vi "tm3samp_09_masterpulse_sequence.vi"() -> ()   [LabVIEW 2011]
panel:
  in  "Interval":dbl=0.5
  out "DCAM Version":string
  out "Library Version":string
  out "Image":u16[][](graph)
  out "Frames Per Second":dbl
  in  "Quit":bool
  out "Error Out":errorcluster {"code" format="%.0x"}
  # "This example will demonstrate how to configure the master pulse and use it for internal trigger capture.  The master pulse signal is also sent to the output trigger in this example."
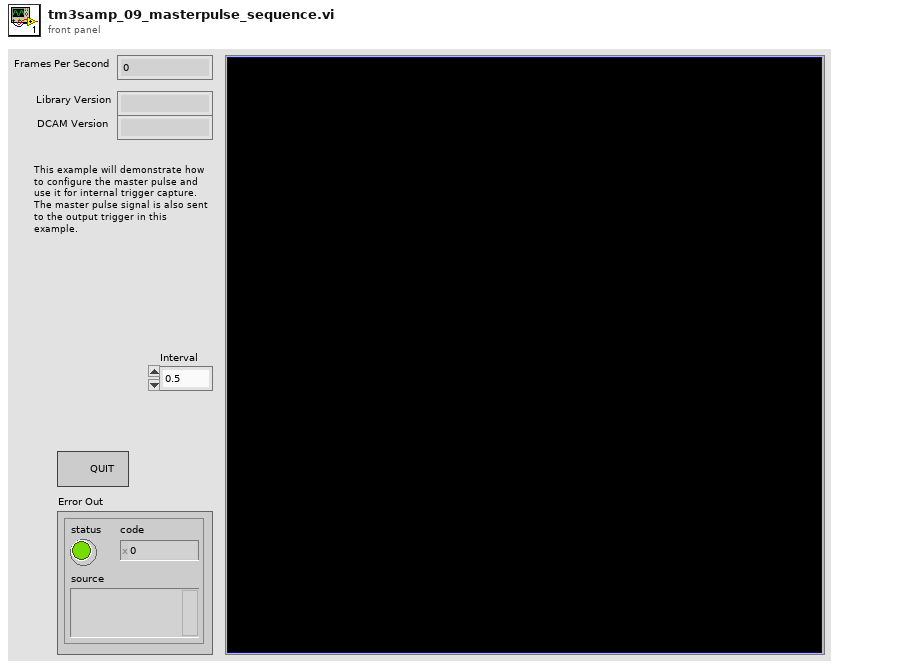
[diagram p1: front panel]
types:
  T1 = cluster{"Capture Library":string, "DCAM-API":string}
  T2 = cluster{"Mode":u32, "Polarity":u32, "Period":dbl, "Delay":dbl}
  T3 = cluster{"Mode":u32, "Source":u32, "Interval":dbl, "Burst":u32}
  T4 = cluster{"height":u32, "width":u32, "datatype":u32}
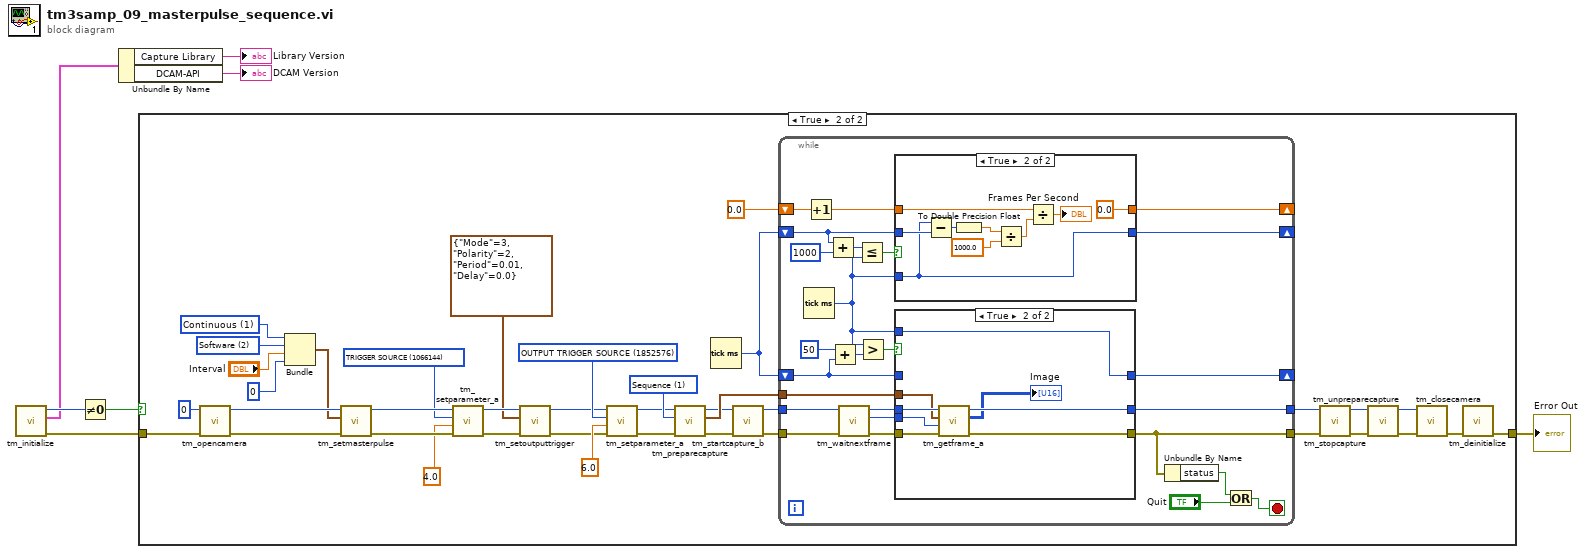
[diagram p0: block diagram]
diagram:
  n1 = call <userlib>:"tm_initialize.vi"() -> ("error out"=w4:errorcluster, "Version Info"=w3:T1, "Number Of Cameras"=w5:u32)  [unwired: 8 in, 1 out]
  n2 = Not Equal To 0?(x=w5) -> (x != 0?=w7:bool)
  n3 = Unbundle By Name(w3) -> ("Capture Library"=→"Library Version":string, "DCAM-API"=→"DCAM Version":string)
  n4 = case shown="True" w7 {
    tunnel: w4 -> [w8 w46]
    tunnel: [w8 w43] -> w6
    frame False {
    }
    frame True {
      w17 = u32 1852576 items=["SENSOR MODE"=4212128, "CCD MODE"=4212384, "READOUT MODE"=4211872, "ACTIVE VIEW INDEX"=4343136, "BITS PER CHANNEL"=4342976, "IMAGE PIXEL TYPE"=4343296, "BINNING"=4215968, "EXPOSURE TIME"=2049184, "CONTRAST GAIN"=3163312, "CONTRAST OFFSET"=3163328, "LIGHT MODE"=2114720, "SENSITIVITY"=2114992, "PHOTON IMAGING MODE"=2115200, "HIGH DYNAMIC RANGE MODE"=3163360, "WHITE BALANCE"=3163568, "TEMPERATURE"=2115232, "TEMPERATURE TARGET"=2115264, "SENSOR COOLER FAN"=2115296, "LINEBUNDLE HEIGHT"=4212192, "MECHANICAL SHUTTER"=2115488, "BACK FOCUS POSITION"=8422304, "TRIGGER CONNECTOR"=1066432, "TRIGGER SOURCE"=1066144, "OUTPUT TRIGGER SOURCE"=1852576, "TRIGGER GLOBAL EXPOSURE"=2049680, "FIRST TRIGGER BEHAVIOR"=2049696, "CHANNEL SYNC"=1852352, "READOUT DIRECTION"=4211904, "PRE HSYNC COUNT"=1852704, "INTERNAL LINE SPEED"=4226000, "INTERNAL LINE INTERVAL"=4226016] ("Parameter")
      w19 = u32 1066144 items=["SENSOR MODE"=4212128, "CCD MODE"=4212384, "READOUT MODE"=4211872, "ACTIVE VIEW INDEX"=4343136, "BITS PER CHANNEL"=4342976, "IMAGE PIXEL TYPE"=4343296, "BINNING"=4215968, "EXPOSURE TIME"=2049184, "CONTRAST GAIN"=3163312, "CONTRAST OFFSET"=3163328, "LIGHT MODE"=2114720, "SENSITIVITY"=2114992, "PHOTON IMAGING MODE"=2115200, "HIGH DYNAMIC RANGE MODE"=3163360, "WHITE BALANCE"=3163568, "TEMPERATURE"=2115232, "TEMPERATURE TARGET"=2115264, "SENSOR COOLER FAN"=2115296, "LINEBUNDLE HEIGHT"=4212192, "MECHANICAL SHUTTER"=2115488, "BACK FOCUS POSITION"=8422304, "TRIGGER CONNECTOR"=1066432, "TRIGGER SOURCE"=1066144, "OUTPUT TRIGGER SOURCE"=1852576, "TRIGGER GLOBAL EXPOSURE"=2049680, "FIRST TRIGGER BEHAVIOR"=2049696, "CHANNEL SYNC"=1852352, "READOUT DIRECTION"=4211904, "PRE HSYNC COUNT"=1852704, "INTERNAL LINE SPEED"=4226000, "INTERNAL LINE INTERVAL"=4226016] ("Parameter")
      w25 = u32 2 items=["External"=1, "Software"=2] ("Source")
      w26 = u32 1 items=["Continuous"=1, "Start"=2, "Burst"=3] ("Mode")
      w34 = 1 items=["Snap", "Sequence"] ("Capture mode")
      n5 = call <userlib>:"tm_opencamera.vi"("error in (no error)"=w46, "Camera Index"=u32 0) -> ("error out"=w27:errorcluster, "Handle out"=w28:u32)  [unwired: 7 in, 1 out]
      n6 = Bundle("Mode"=w26, "Source"=w25, "Interval"="Interval", "Burst"=u32 0) -> (w23:T3)  [unwired: 1 in]
      n7 = call <userlib>:"tm_setmasterpulse.vi"("error in (no error)"=w27, "Parameters"=w23, "Handle in"=w28) -> ("error out"=w20:errorcluster, "Handle out"=w21:u32)  [unwired: 7 in]
      n8 = call <userlib>:"tm_setparameter_a.vi"("error in (no error)"=w20, "Value in"=4.0, "Parameter"=w19, "Handle in"=w21) -> ("error out"=w12:errorcluster, "Handle out"=w13:u32)  [unwired: 6 in]
      n9 = call <userlib>:"tm_setoutputtrigger.vi"("error in (no error)"=w12, "Parameters"=T2 {"Mode"=3, "Polarity"=2, "Period"=0.01, "Delay"=0.0}, "Handle in"=w13) -> ("error out"=w10:errorcluster, "Handle out"=w11:u32)  [unwired: 7 in]
      n10 = call <userlib>:"tm_setparameter_a.vi"("error in (no error)"=w10, "Value in"=6.0, "Parameter"=w17, "Handle in"=w11) -> ("error out"=w14:errorcluster, "Handle out"=w15:u32)  [unwired: 6 in]
      n11 = call <userlib>:"tm_preparecapture.vi"("error in (no error)"=w14, "Capture mode"=w34, "Handle in"=w15) -> ("error out"=w31:errorcluster, "Buffer Info"=w33:T4, "Handle out"=w32:u32)  [unwired: 5 in, 1 out]
      n12 = Tick Count (ms)() -> (millisecond timer value=w29:u32)
      n13 = call <userlib>:"tm_startcapture_b.vi"("error in (no error)"=w31, "Handle in"=w32) -> ("error out"=w35:errorcluster, "Handle out"=w36:u32)  [unwired: 8 in]
      n14 = while {
        tunnel: [w50] -> w39
        tunnel: [w51] -> w40
        tunnel: w33 -> [w48]
        tunnel: w36 -> [w68]
        tunnel: w35 -> [w69]
        shift-right: [w66] -> _
        shift-left: w29 -> [w63]
        shift-right: [w67] -> _
        shift-left: 0.0 -> [w60]
        shift-right: [w49] -> _
        shift-left: w29 -> [w52]
        stop <- w47 stop-if-true
        n15 = Tick Count (ms)() -> (millisecond timer value=w53:u32)
        n16 = Increment(x=w60) -> (x+1=w61:dbl)
        n17 = Add(x=w63, y=u32 1000) -> (x+y=w65:u32)
        n18 = Add(x=u32 50, y=w52) -> (x+y=w55:u32)
        n19 = call <userlib>:"tm_waitnextframe.vi"("error in (no error)"=w69, "Handle in"=w68) -> ("error out"=w58:errorcluster, "Frame Index"=w57:i32, "Handle out"=w59:u32)  [unwired: 6 in, 1 out]
        n20 = Less Or Equal?(x=w65, y=w53) -> (x <= y?=w62:bool)
        n21 = Greater?(x=w53, y=w55) -> (0:w54:bool)
        n22 = case shown="True" w62 {
          tunnel: w63 -> [w84 w87]
          tunnel: [w84 w85] -> w66
          tunnel: w61 -> [w83 w91]
          tunnel: w53 -> [_ w85]
          tunnel: [w83 0.0] -> w67
          frame False {
          }
          frame True {
            n23 = Subtract(x=w85, y=w87) -> (x-y=w86:u32)
            n24 = To Double Precision Float(number=w86) -> (double precision float=w93:dbl)
            n25 = Divide(x=w93, y=1000.0) -> (x/y=w90:dbl)
            n26 = Divide(x=w91, y=w90) -> (x/y=→"Frames Per Second":dbl)
          }
        }
        n27 = case shown="True" w54 {
          tunnel: w59 -> [w74 w82]
          tunnel: w58 -> [w73 w81]
          tunnel: w57 -> [_ w80]
          tunnel: w52 -> [w72 _]
          tunnel: w53 -> [_ w79]
          tunnel: [w74 w76] -> w50
          tunnel: [w73 w77] -> w51
          tunnel: [w72 w79] -> w49
          tunnel: w48 -> [_ w78]
          frame False {
          }
          frame True {
            n28 = call <userlib>:"tm_getframe_a.vi"("error in (no error)"=w81, "Frame Index"=w80, "Buffer Info"=w78, "Handle in"=w82) -> ("error out"=w77:errorcluster, "Data 16"=→"Image":u16[][], "Handle out"=w76:u32)  [unwired: 3 in, 2 out]
          }
        }
        n29 = Unbundle By Name(w51) -> ("status"=w71:bool)
        n30 = Or(x=w71, y="Quit") -> (x .or. y?=w47:bool)
      }
      n31 = call <userlib>:"tm_stopcapture.vi"("error in (no error)"=w40, "Handle in"=w39) -> ("error out"=w37:errorcluster, "Handle out"=w38:u32)  [unwired: 8 in]
      n32 = call <userlib>:"tm_unpreparecapture.vi"("error in (no error)"=w37, "Handle in"=w38) -> ("error out"=w42:errorcluster, "Handle out"=w41:u32)  [unwired: 8 in]
      n33 = call <userlib>:"tm_closecamera.vi"("error in (no error)"=w42, "Handle in"=w41) -> ("error out"=w44:errorcluster)  [unwired: 9 in]
      n34 = call <userlib>:"tm_deinitialize.vi"("error in (no error)"=w44) -> ("error out"=w43:errorcluster)  [unwired: 10 in]
    }
  }
  "Error Out" <- w6
